vi "array_ascii.vi"() -> ()   [LabVIEW 2025]
panel:
  out "appended array":dbl[](array[numeric])
  out "string":string
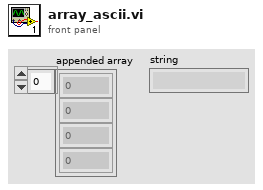
[diagram p1: front panel]
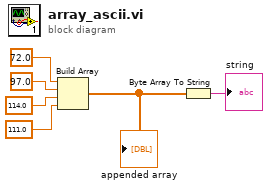
[diagram p0: block diagram]
diagram:
  n1 = Build Array(72.0 ("element"), 97.0 ("element"), 114.0 ("element"), 111.0 ("element")) -> (w1:dbl[])
  "appended array" <- w1
  n2 = Byte Array To String(unsigned byte array=w1) -> (string=→"string":string)
